vi "PR_COM_Labview_Demo.vi"() -> ()   [LabVIEW 2017]
uses:
  D:/Projects/GUI/Power Rider Wrapper/PowerRiderDLLWrapper.dll
  PowerRiderDLLWrapper.dll
panel:
  in  "VISA res_in":refnum<visa-resource-name>
  in  "baud rate":u32(ring)=19200 items=["921600"=921600, "460800"=460800, "256000"=256000, "115200"=115200, "57600"=57600, "38400"=38400, "19200"=19200, "14400"=14400, "9600"=9600, "2400"=2400, "1200"=1200]
  in  "Status Enum":enum16{"OFF", "ON", "ERROR", "FOREVER OFF"}(ring)
  in  "TripType Enum":T1(ring)
  in  "address":u16=85
  in  "Dst add":u16=16
  out "CommIcon":bool
  in  "String":string
  # "Power Rider Demo"
  # "Serial COM interface"
  # "ver 1.0"
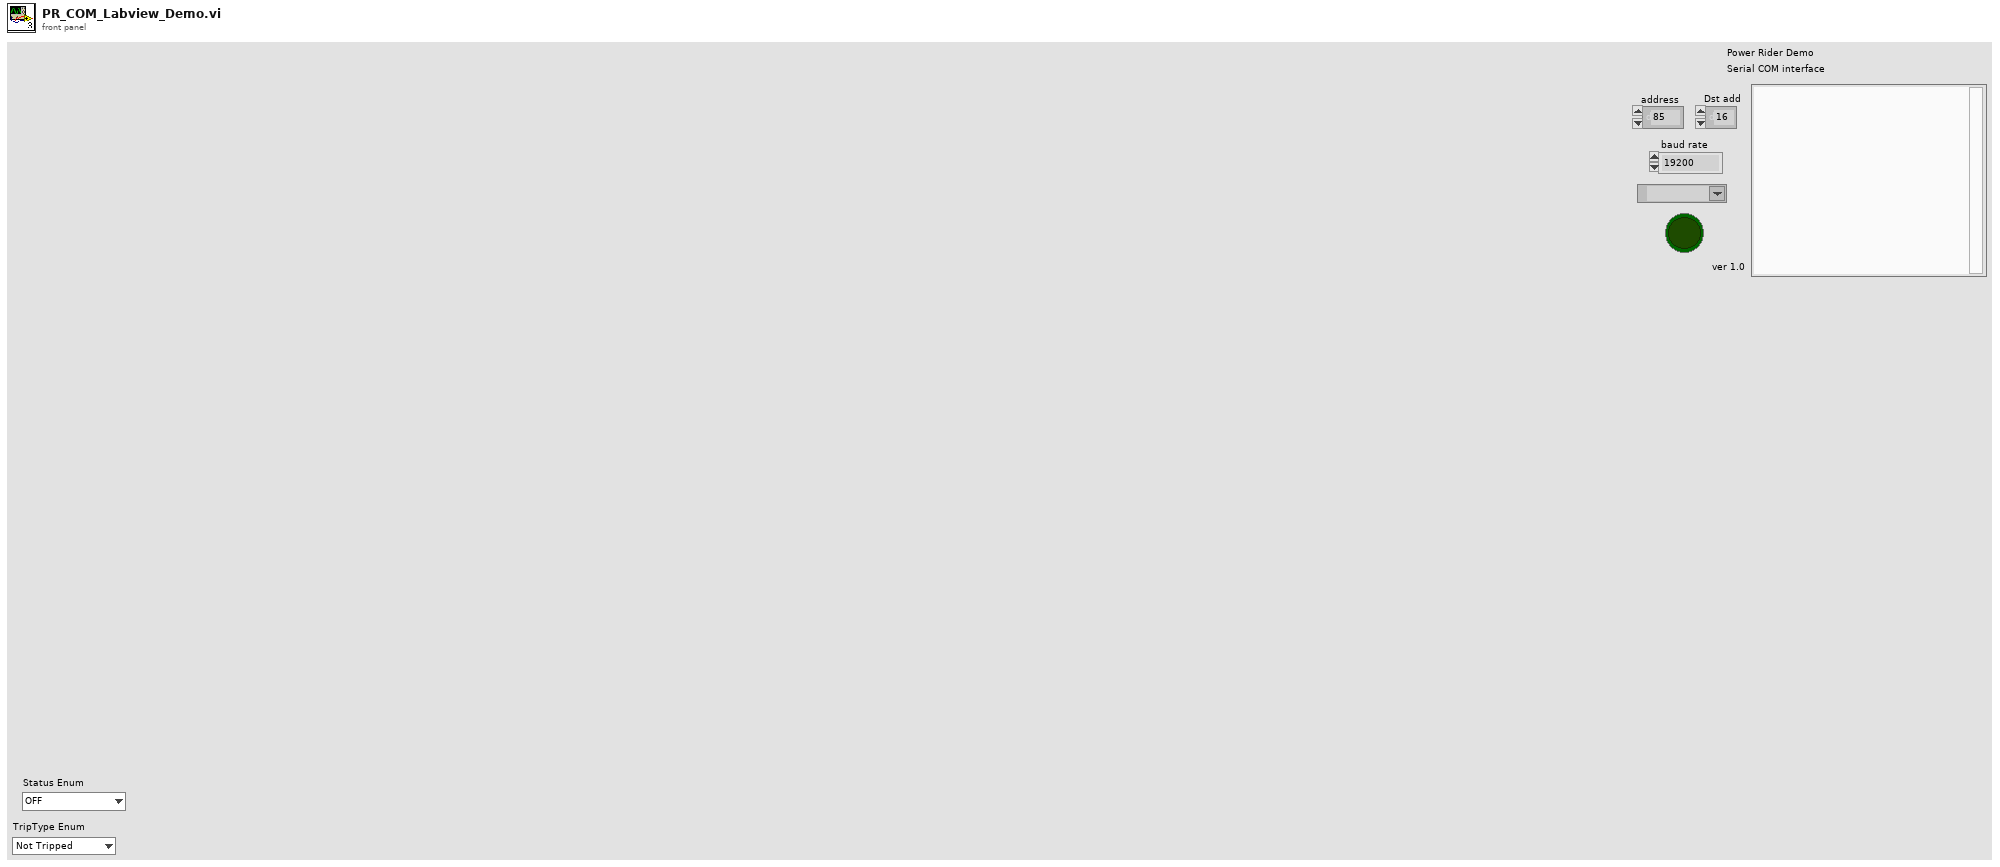
[diagram p1: front panel]
types:
  T1 = enum16{"Not Tripped", "SW Tripped", "Hard Short", "MAX SW Tripped"}
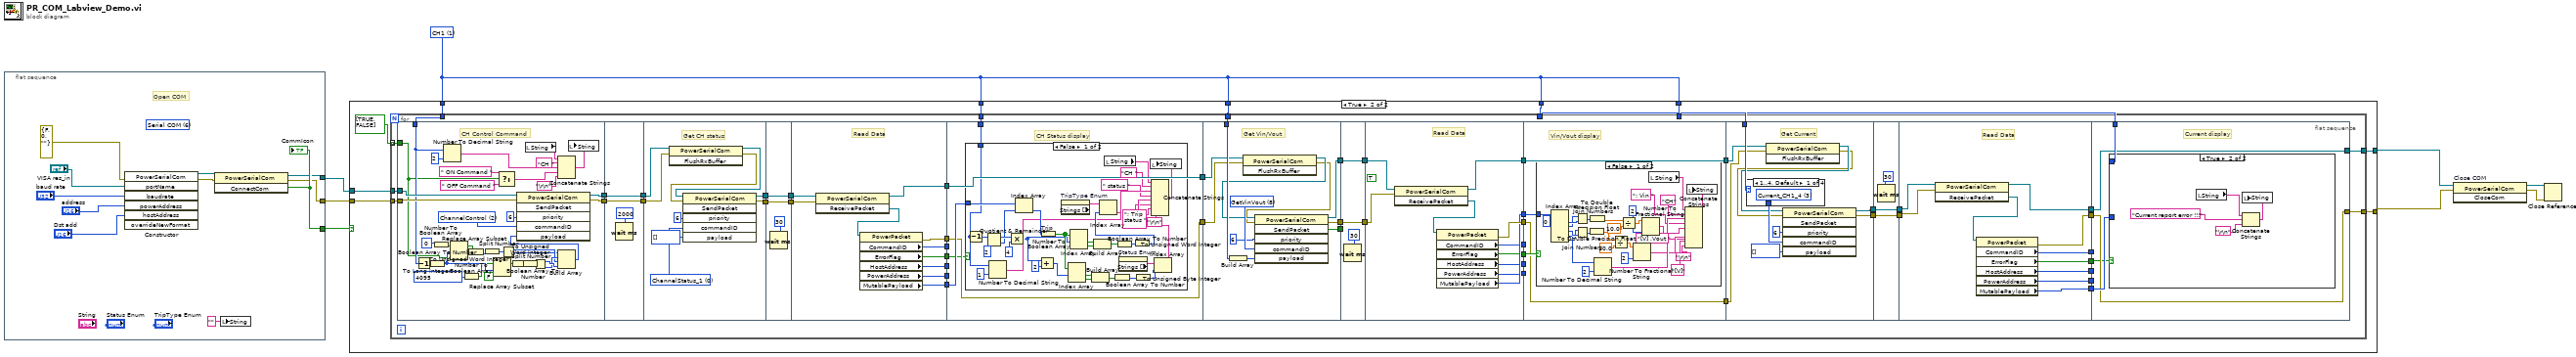
[diagram p0: block diagram]
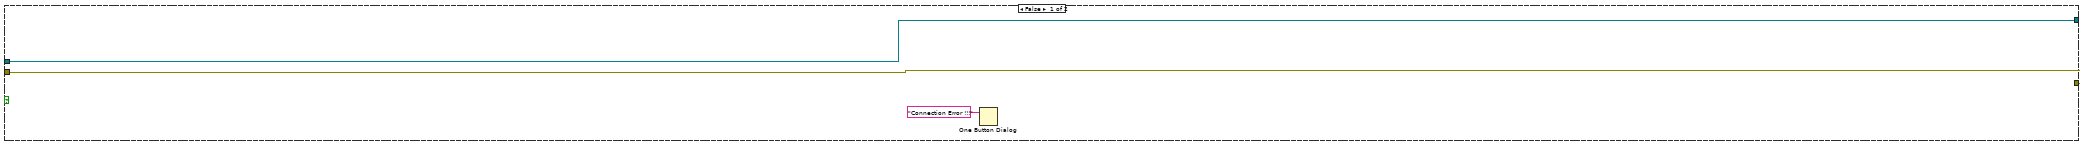
[diagram p2: hidden frame]
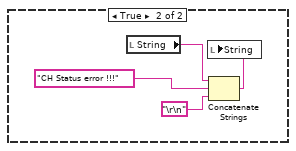
[diagram p3: hidden frame]
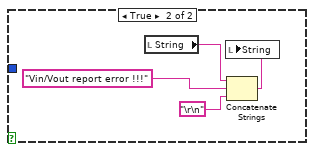
[diagram p4: hidden frame]
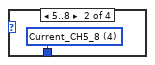
[diagram p5: hidden frame]
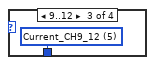
[diagram p6: hidden frame]
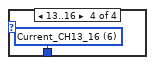
[diagram p7: hidden frame]
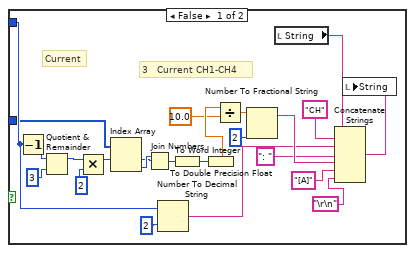
[diagram p8: hidden frame]
diagram:
  w5 = u8 1 items=["CH1"=1, "CH2"=2, "CH3"=3, "CH4"=4, "CH5"=5, "CH6"=6, "CH7"=7, "CH8"=8, "CH9"=9, "CH10"=10, "CH11"=11, "CH12"=12, "CH13"=13, "CH14"=14, "CH15"=15, "CH16"=16] ("Select CH #")
  n1 = flat-sequence {
    tunnel: [w18] -> w8
    tunnel: [w17] -> w2
    tunnel: [w16] -> w1
    frame #0 {
      (unwired) u16 6 items=["CANalystII"=2, "TCP Client"=3, "TCP Server"=4, "UDP Client"=5, "Serial COM"=6, "CAN Kvaser"=7] ("COMType 2")
      # "Open COM"
      n2 = constructor class="PowerSerialCom"(error in=errorcluster {"status"=FALSE, "code"=0, "source"=""} ("error out"), "portName"="VISA res_in", "baudrate"="baud rate", "powerAddress"="address", "hostAddress"="Dst add") -> (reference out=w10:refnum<k24>, error out=w9:errorcluster)  [unwired: 3 in, 6 out]
      n3 = invoke class="PowerSerialCom" method="ConnectCom"(reference=w10, error in=w9) -> (reference out=w16:refnum<k24>, error out=w17:errorcluster, "ConnectCom"=w18:bool)  [unwired: 1 in]
      "CommIcon" <- w18
      n4 = local write "String"("" ("String")) -> ()
    }
  }
  n5 = case shown="True" w8 {
    tunnel: w1 -> [w21 w27]
    tunnel: w2 -> [w22 w26]
    tunnel: w5 -> [_ w32]
    tunnel: w5 -> [_ w31]
    tunnel: w5 -> [_ w30]
    tunnel: w5 -> [_ w29]
    tunnel: w5 -> [_ w28]
    tunnel: [w21 w25] -> w4
    tunnel: [w22 w24] -> w3
    frame False {
      n6 = One Button Dialog(message="Connection Error !!!") -> ()  [unwired: 1 in, 1 out]
    }
    frame True {
      n7 = for {
        tunnel: w32 -> [w33]
        tunnel: w31 -> [w73]
        tunnel: w30 -> [w72]
        tunnel: w29 -> [w71]
        tunnel: w28 -> [w34]
        tunnel: w27 -> [w70]
        tunnel: w26 -> [w69]
        tunnel: [w68] -> w25
        tunnel: [w67] -> w24
        tunnel: bool[] [TRUE, FALSE] -> [w66] mode=indexing
        n8 = flat-sequence {
          tunnel: w69 -> [w98]
          tunnel: [w100] -> w84
          tunnel: [w99] -> w83
          tunnel: w34 -> [w93]
          tunnel: w70 -> [w97]
          tunnel: w66 -> [w89]
          tunnel: w84 -> [w122]
          tunnel: [w122] -> w82
          tunnel: w83 -> [w121]
          tunnel: [w121] -> w81
          tunnel: [w128] -> w65
          tunnel: [w127] -> w63
          tunnel: w82 -> [w126]
          tunnel: w81 -> [w125]
          tunnel: w65 -> [w134]
          tunnel: [w134] -> w64
          tunnel: w63 -> [w133]
          tunnel: [w133] -> w62
          tunnel: w64 -> [w141]
          tunnel: w62 -> [w142]
          tunnel: [w144] -> w80
          tunnel: [w143] -> w79
          tunnel: [w139] -> w78
          tunnel: [w138] -> w47
          tunnel: [w137] -> w46
          tunnel: [w136] -> w45
          tunnel: [w135] -> w44
          tunnel: w80 -> [w147]
          tunnel: w79 -> [w149]
          tunnel: w78 -> [w148]
          tunnel: [w148] -> w77
          tunnel: [w147] -> w76
          tunnel: w33 -> [w146]
          tunnel: w47 -> [w145]
          tunnel: w46 -> [_]
          tunnel: w45 -> [_]
          tunnel: w44 -> [_]
          tunnel: w77 -> [w191]
          tunnel: w76 -> [w189]
          tunnel: w73 -> [w193]
          tunnel: [w195] -> w61
          tunnel: [w194] -> w60
          tunnel: [w192] -> w43
          tunnel: w61 -> [w201]
          tunnel: [w201] -> w58
          tunnel: w60 -> [w200]
          tunnel: [w200] -> w56
          tunnel: w43 -> [_]
          tunnel: [w210] -> w59
          tunnel: w58 -> [w208]
          tunnel: [w207] -> w57
          tunnel: w56 -> [w209]
          tunnel: [w211] -> w55
          tunnel: [w205] -> w42
          tunnel: [w204] -> w41
          tunnel: [w203] -> w40
          tunnel: [w202] -> w39
          tunnel: w59 -> [w215]
          tunnel: [w214] -> w75
          tunnel: w57 -> [w214]
          tunnel: w55 -> [w212]
          tunnel: [w212] -> w74
          tunnel: w42 -> [_]
          tunnel: w41 -> [w213]
          tunnel: w40 -> [_]
          tunnel: w39 -> [_]
          tunnel: w72 -> [w256]
          tunnel: w75 -> [w251]
          tunnel: w74 -> [w250]
          tunnel: [w253] -> w54
          tunnel: [w252] -> w53
          tunnel: w54 -> [w264]
          tunnel: [w264] -> w52
          tunnel: w53 -> [w263]
          tunnel: [w263] -> w50
          tunnel: w52 -> [w272]
          tunnel: [w273] -> w51
          tunnel: w50 -> [w271]
          tunnel: [w269] -> w49
          tunnel: [w274] -> w48
          tunnel: [w268] -> w38
          tunnel: [w267] -> w37
          tunnel: [w266] -> w36
          tunnel: [w265] -> w35
          tunnel: w51 -> [w276]
          tunnel: w49 -> [w277]
          tunnel: w71 -> [w279]
          tunnel: w48 -> [w278]
          tunnel: [w277] -> w68
          tunnel: [w276] -> w67
          tunnel: w38 -> [w275]
          tunnel: w37 -> [_]
          tunnel: w36 -> [_]
          tunnel: w35 -> [_]
          frame #0 {
            w101 = u8 2 items=["ChannelStatus_1"=0, "ChannelControl"=2, "Current_CH1_4"=3, "Current_CH5_8"=4, "Current_CH9_12"=5, "Current_CH13_16"=6, "GetVinVout"=8, "Version_BoardType"=9, "SystemTemp"=10, "SystemParameter"=11, "ChannelParameter"=12, "GetTripEvent"=15, "LogFile"=18, "Configuration"=19, "ProductionData"=20, "BIT"=33, "DiscretePorts"=34, "SerialNumber"=36, "OffsetMeasurement"=37, "PartNumber"=39, "ChannelCombinedStatus_1_CH1_8"=40, "ChannelCombinedStatus_2_CH9_12"=41, "PlotData"=45, "PlotCommand"=46, "InternalData"=47, "KeepAlive"=234, "WakeUp"=250] ("commandID")
            # "CH Control Command"
            n9 = Decrement(x=w93) -> (x-1=w102:u8)
            n10 = To Long Integer(number=w102) -> (32bit integer=w108:i32)
            n11 = Number To Boolean Array(number=u16 0 ("element")) -> (Boolean array=w104:bool[])
            n12 = Number To Decimal String(number=w93, width (-)=i16 2) -> (decimal integer string=w90:string)
            n13 = Replace Array Subset(array=w104, new element=w89, index=w108) -> (w105:bool[])
            n14 = Number To Boolean Array(number=u16 4095 ("mask")) -> (Boolean array=w107:bool[])
            n15 = Boolean Array To Number(Boolean array=w105) -> (number=w106:u32)
            n16 = To Unsigned Word Integer(number=w106) -> (unsigned 16bit integer=w113:u16)
            n17 = Replace Array Subset(array=w107, new element=FALSE ("new element/subarray"), index=w108) -> (w103:bool[])
            n18 = Select(t=" ON Command " ("string"), s=w89, f=" OFF Command " ("string")) -> (s? t:f=w86:string)
            n19 = Split Number(x=w113) -> (hi(x)=w117:u8, lo(x)=w116:u8)
            n20 = Boolean Array To Number(Boolean array=w103) -> (number=w112:u32)
            n21 = To Unsigned Word Integer(number=w112) -> (unsigned 16bit integer=w115:u16)
            n22 = local read "String"() -> (w95:string)
            n23 = Split Number(x=w115) -> (hi(x)=w119:u8, lo(x)=w118:u8)
            n24 = Concatenate Strings(w95, "CH " ("string"), w90, w86, "\r\n") -> (w94:string)
            n25 = Build Array(w116, w118, w117, w119) -> (w114:u8[])
            n26 = invoke class="PowerSerialCom" method="SendPacket"(reference=w97, error in=w98, "priority"=u8 6, "commandID"=w101, "payload"=w114) -> (reference out=w100:refnum<k24>, error out=w99:errorcluster)  [unwired: 1 in, 4 out]
            n27 = local write "String"(w94) -> ()
          }
          frame #1 {
            n28 = Wait (ms)(milliseconds to wait=u32 2000) -> ()  [unwired: 1 out]
          }
          frame #2 {
            w131 = u8 0 items=["ChannelStatus_1"=0, "ChannelControl"=2, "Current_CH1_4"=3, "Current_CH5_8"=4, "Current_CH9_12"=5, "Current_CH13_16"=6, "GetVinVout"=8, "Version_BoardType"=9, "SystemTemp"=10, "SystemParameter"=11, "ChannelParameter"=12, "GetTripEvent"=15, "LogFile"=18, "Configuration"=19, "ProductionData"=20, "BIT"=33, "DiscretePorts"=34, "SerialNumber"=36, "OffsetMeasurement"=37, "PartNumber"=39, "ChannelCombinedStatus_1_CH1_8"=40, "ChannelCombinedStatus_2_CH9_12"=41, "PlotData"=45, "PlotCommand"=46, "InternalData"=47, "KeepAlive"=234, "WakeUp"=250] ("commandID")
            # "Get CH status"
            n29 = invoke class="PowerSerialCom" method="FlushRxBuffer"(reference=w126, error in=w125) -> (reference out=w123:refnum<k24>, error out=w124:errorcluster)  [unwired: 1 in, 1 out]
            n30 = invoke class="PowerSerialCom" method="SendPacket"(reference=w123, error in=w124, "priority"=u8 6, "commandID"=w131, "payload"=u8[] []) -> (reference out=w127:refnum<k24>, error out=w128:errorcluster)  [unwired: 1 in, 4 out]
          }
          frame #3 {
            n31 = Wait (ms)(milliseconds to wait=u32 30) -> ()  [unwired: 1 out]
          }
          frame #4 {
            # "Read Data"
            n32 = invoke class="PowerSerialCom" method="ReceivePacket"(reference=w142, error in=w141) -> (reference out=w139:refnum<k24>, "ReceivePacket"=w140:refnum<k24>)  [unwired: 1 in, 1 out]
            n33 = property class="PowerPacket"(reference=w140) -> (error out=w144:errorcluster, "CommandID"=w137:u8, "ErrorFlag"=w138:bool, "HostAddress"=w136:u8, "PowerAddress"=w135:u8, "MutablePayload"=w143:u8[])  [unwired: 1 in, 1 out]
          }
          frame #5 {
            # "CH Status display"
            n34 = case shown="False" w145 {
              tunnel: w149 -> [w156 _]
              tunnel: w146 -> [w153 _]
              frame False {
                n35 = Decrement(x=w153) -> (x-1=w150:u8)
                n36 = Quotient & Remainder(x=w150, y=2) -> (x-y*floor(x/y)=w166:i32, floor(x/y)=w165:i32)
                n37 = Number To Decimal String(number=w153, width (-)=i16 1) -> (decimal integer string=w169:string)
                n38 = Multiply(x=w166, y=u8 4) -> (x*y=w164:i32)
                n39 = Index Array(array=w156, index=w165) -> (element=w171:u8)
                n40 = Add(x=w164, y=u8 2) -> (x+y=w163:i32)
                n41 = Number To Boolean Array "Trip"(number=w171) -> (Boolean array=w170:bool[])
                n42 = property on="TripType Enum" class="Enum (strict)"() -> ("Strings []"=w180:string[])  [unwired: 2 in, 2 out]
                n43 = Index Array(array=w170, index #1=w163) -> (element #1=w179:bool, element #2=w178:bool)  [unwired: 1 in]
                n44 = Index Array(array=w170, index #1=w164) -> (element #1=w176:bool, element #2=w177:bool)  [unwired: 1 in]
                n45 = Build Array(w179, w178) -> (w175:bool[])
                n46 = Build Array(w176, w177) -> (w174:bool[])
                n47 = local read "String"() -> (w152:string)
                n48 = Boolean Array To Number(Boolean array=w175) -> (number=w173:u32)
                n49 = Boolean Array To Number(Boolean array=w174) -> (number=w172:u32)
                n50 = property on="Status Enum" class="Enum (strict)"() -> ("Strings []"=w181:string[])  [unwired: 2 in, 2 out]
                n51 = To Unsigned Word Integer(number=w172) -> (unsigned 16bit integer=w182:u16)
                n52 = Index Array(array=w180, index=w182) -> (element=w168:string)
                n53 = To Unsigned Byte Integer(number=w173) -> (unsigned 8bit integer=w183:u8)
                n54 = Index Array(array=w181, index=w183) -> (element=w167:string)
                n55 = Concatenate Strings(w152, "CH " ("string"), w169, " status ", w167, "; Trip status ", w168, "\r\n") -> (w155:string)
                n56 = local write "String"(w155) -> ()
              }
              frame True {
                n57 = local read "String"() -> (w186:string)
                n58 = Concatenate Strings(w186, "CH Status error !!!" ("string"), "\r\n") -> (w187:string)
                n59 = local write "String"(w187) -> ()
              }
            }
          }
          frame #6 {
            w197 = u8 8 items=["ChannelStatus_1"=0, "ChannelControl"=2, "Current_CH1_4"=3, "Current_CH5_8"=4, "Current_CH9_12"=5, "Current_CH13_16"=6, "GetVinVout"=8, "Version_BoardType"=9, "SystemTemp"=10, "SystemParameter"=11, "ChannelParameter"=12, "GetTripEvent"=15, "LogFile"=18, "Configuration"=19, "ProductionData"=20, "BIT"=33, "DiscretePorts"=34, "SerialNumber"=36, "OffsetMeasurement"=37, "PartNumber"=39, "ChannelCombinedStatus_1_CH1_8"=40, "ChannelCombinedStatus_2_CH9_12"=41, "PlotData"=45, "PlotCommand"=46, "InternalData"=47, "KeepAlive"=234, "WakeUp"=250] ("commandID")
            # "Get Vin/Vout"
            n60 = Build Array(w193) -> (w198:u8[])
            n61 = invoke class="PowerSerialCom" method="FlushRxBuffer"(reference=w191, error in=w189) -> (reference out=w190:refnum<k24>, error out=w188:errorcluster)  [unwired: 1 in, 1 out]
            n62 = invoke class="PowerSerialCom" method="SendPacket"(reference=w190, error in=w188, "priority"=u8 6, "commandID"=w197, "payload"=w198) -> (reference out=w195:refnum<k24>, error out=w194:errorcluster, "SendPacket"=w192:bool)  [unwired: 1 in, 3 out]
          }
          frame #7 {
            n63 = Wait (ms)(milliseconds to wait=u32 30) -> ()  [unwired: 1 out]
          }
          frame #8 {
            (unwired) TRUE
            # "Read Data"
            n64 = invoke class="PowerSerialCom" method="ReceivePacket"(reference=w208, error in=w209) -> (reference out=w207:refnum<k24>, "ReceivePacket"=w206:refnum<k24>)  [unwired: 1 in, 1 out]
            n65 = property class="PowerPacket"(reference=w206) -> (error out=w211:errorcluster, "CommandID"=w205:u8, "ErrorFlag"=w204:bool, "HostAddress"=w203:u8, "PowerAddress"=w202:u8, "MutablePayload"=w210:u8[])  [unwired: 1 in, 1 out]
          }
          frame #9 {
            # "Vin/Vout display"
            n66 = case shown="False" w213 {
              tunnel: w215 -> [w219 _]
              frame False {
                n67 = Index Array(array=w219, index #1=0 ("index")) -> (element #1=w241:u8, element #2=w240:u8, element #3=w239:u8, element #4=w238:u8, element #5=w235:u8)  [unwired: 4 in]
                n68 = Join Numbers(hi=w240, lo=w241) -> ((hi.lo)=w242:u16)
                n69 = Join Numbers(hi=w238, lo=w239) -> ((hi.lo)=w243:u16)
                n70 = To Double Precision Float(number=w243) -> (double precision float=w236:dbl)
                n71 = To Double Precision Float(number=w242) -> (double precision float=w237:dbl)
                n72 = Number To Decimal String(number=w235, width (-)=i16 2) -> (decimal integer string=w234:string)
                n73 = Divide(x=w236, y=10.0) -> (x/y=w231:dbl)
                n74 = Divide(x=w237, y=10.0) -> (x/y=w233:dbl)
                n75 = Number To Fractional String(number=w231, precision (6)=i16 2) -> (F-format string=w230:string)  [unwired: 2 in]
                n76 = Number To Fractional String(number=w233, precision (6)=i16 2) -> (F-format string=w232:string)  [unwired: 2 in]
                n77 = local read "String"() -> (w217:string)
                n78 = Concatenate Strings(w217, "CH" ("string"), w234, ": Vin " ("string"), w232, "[V] ,Vout " ("string"), w230, "[V]" ("string"), "\r\n") -> (w218:string)
                n79 = local write "String"(w218) -> ()
              }
              frame True {
                n80 = local read "String"() -> (w246:string)
                n81 = Concatenate Strings(w246, "Vin/Vout report error !!!" ("string"), "\r\n") -> (w247:string)
                n82 = local write "String"(w247) -> ()
              }
            }
          }
          frame #10 {
            # "Get Current"
            n83 = case shown="1..4, Default" w256 {
              tunnel: [w258 w259 w260 w261] -> w257
              frame 1..4, Default {
                w258 = u8 3 items=["ChannelStatus_1"=0, "ChannelControl"=2, "Current_CH1_4"=3, "Current_CH5_8"=4, "Current_CH9_12"=5, "Current_CH13_16"=6, "GetVinVout"=8, "Version_BoardType"=9, "SystemTemp"=10, "SystemParameter"=11, "ChannelParameter"=12, "GetTripEvent"=15, "LogFile"=18, "Configuration"=19, "ProductionData"=20, "BIT"=33, "DiscretePorts"=34, "SerialNumber"=36, "OffsetMeasurement"=37, "PartNumber"=39, "ChannelCombinedStatus_1_CH1_8"=40, "ChannelCombinedStatus_2_CH9_12"=41, "PlotData"=45, "PlotCommand"=46, "InternalData"=47, "KeepAlive"=234, "WakeUp"=250] ("commandID")
              }
              frame 5..8 {
                w259 = u8 4 items=["ChannelStatus_1"=0, "ChannelControl"=2, "Current_CH1_4"=3, "Current_CH5_8"=4, "Current_CH9_12"=5, "Current_CH13_16"=6, "GetVinVout"=8, "Version_BoardType"=9, "SystemTemp"=10, "SystemParameter"=11, "ChannelParameter"=12, "GetTripEvent"=15, "LogFile"=18, "Configuration"=19, "ProductionData"=20, "BIT"=33, "DiscretePorts"=34, "SerialNumber"=36, "OffsetMeasurement"=37, "PartNumber"=39, "ChannelCombinedStatus_1_CH1_8"=40, "ChannelCombinedStatus_2_CH9_12"=41, "PlotData"=45, "PlotCommand"=46, "InternalData"=47, "KeepAlive"=234, "WakeUp"=250] ("commandID")
              }
              frame 9..12 {
                w260 = u8 5 items=["ChannelStatus_1"=0, "ChannelControl"=2, "Current_CH1_4"=3, "Current_CH5_8"=4, "Current_CH9_12"=5, "Current_CH13_16"=6, "GetVinVout"=8, "Version_BoardType"=9, "SystemTemp"=10, "SystemParameter"=11, "ChannelParameter"=12, "GetTripEvent"=15, "LogFile"=18, "Configuration"=19, "ProductionData"=20, "BIT"=33, "DiscretePorts"=34, "SerialNumber"=36, "OffsetMeasurement"=37, "PartNumber"=39, "ChannelCombinedStatus_1_CH1_8"=40, "ChannelCombinedStatus_2_CH9_12"=41, "PlotData"=45, "PlotCommand"=46, "InternalData"=47, "KeepAlive"=234, "WakeUp"=250] ("commandID")
              }
              frame 13..16 {
                w261 = u8 6 items=["ChannelStatus_1"=0, "ChannelControl"=2, "Current_CH1_4"=3, "Current_CH5_8"=4, "Current_CH9_12"=5, "Current_CH13_16"=6, "GetVinVout"=8, "Version_BoardType"=9, "SystemTemp"=10, "SystemParameter"=11, "ChannelParameter"=12, "GetTripEvent"=15, "LogFile"=18, "Configuration"=19, "ProductionData"=20, "BIT"=33, "DiscretePorts"=34, "SerialNumber"=36, "OffsetMeasurement"=37, "PartNumber"=39, "ChannelCombinedStatus_1_CH1_8"=40, "ChannelCombinedStatus_2_CH9_12"=41, "PlotData"=45, "PlotCommand"=46, "InternalData"=47, "KeepAlive"=234, "WakeUp"=250] ("commandID")
              }
            }
            n84 = invoke class="PowerSerialCom" method="FlushRxBuffer"(reference=w251, error in=w250) -> (reference out=w249:refnum<k24>, error out=w248:errorcluster)  [unwired: 1 in, 1 out]
            n85 = invoke class="PowerSerialCom" method="SendPacket"(reference=w249, error in=w248, "priority"=u8 6, "commandID"=w257, "payload"=u8[] []) -> (reference out=w252:refnum<k24>, error out=w253:errorcluster)  [unwired: 1 in, 4 out]
          }
          frame #11 {
            n86 = Wait (ms)(milliseconds to wait=u32 30) -> ()  [unwired: 1 out]
          }
          frame #12 {
            # "Read Data"
            n87 = invoke class="PowerSerialCom" method="ReceivePacket"(reference=w271, error in=w272) -> (reference out=w269:refnum<k24>, "ReceivePacket"=w270:refnum<k24>)  [unwired: 1 in, 1 out]
            n88 = property class="PowerPacket"(reference=w270) -> (error out=w273:errorcluster, "CommandID"=w265:u8, "ErrorFlag"=w268:bool, "HostAddress"=w267:u8, "PowerAddress"=w266:u8, "MutablePayload"=w274:u8[])  [unwired: 1 in, 1 out]
          }
          frame #13 {
            # "Current display"
            n89 = case shown="True" w275 {
              tunnel: w279 -> [w284 _]
              tunnel: w278 -> [w283 _]
              frame False {
                # "3   Current CH1-CH4"
                # "Current"
                n90 = Decrement(x=w284) -> (x-1=w285:u8)
                n91 = Quotient & Remainder(x=w285, y=u8 3) -> (x-y*floor(x/y)=w299:u8)  [unwired: 1 out]
                n92 = Multiply(x=w299, y=u8 2) -> (x*y=w298:u8)
                n93 = Index Array(array=w283, index #1=w298) -> (element #1=w296:u8, element #2=w297:u8)  [unwired: 1 in]
                n94 = Join Numbers(hi=w297, lo=w296) -> ((hi.lo)=w300:u16)
                n95 = Number To Decimal String(number=w284, width (-)=i16 2) -> (decimal integer string=w294:string)
                n96 = To Word Integer(number=w300) -> (16bit integer=w302:i16)
                n97 = To Double Precision Float(number=w302) -> (double precision float=w301:dbl)
                n98 = Divide(x=w301, y=10.0) -> (x/y=w295:dbl)
                n99 = Number To Fractional String(number=w295, precision (6)=i16 2) -> (F-format string=w303:string)  [unwired: 2 in]
                n100 = local read "String"() -> (w280:string)
                n101 = Concatenate Strings(w280, "CH" ("string"), w294, ": " ("string"), w303, "[A]" ("string"), "\r\n") -> (w282:string)
                n102 = local write "String"(w282) -> ()
              }
              frame True {
                n103 = local read "String"() -> (w306:string)
                n104 = Concatenate Strings(w306, "Current report error !!!" ("string"), "\r\n") -> (w307:string)
                n105 = local write "String"(w307) -> ()
              }
            }
          }
        }
      }
    }
  }
  n106 = invoke on="Close COM" class="PowerSerialCom" method="CloseCom"(reference=w4, error in=w3) -> (reference out=w7:refnum<k24>, error out=w6:errorcluster)  [unwired: 1 in, 1 out]
  n107 = Close Reference(reference=w7, error in (no error)=w6) -> ()  [unwired: 1 out]
